vi "Comm String Flush Port.vi"(0 "niDTS Comm Telnet in":refnum<class "niDTS Comm Telnet.lvclass">, 7 "Read Data (F)":bool, 9 "Log Data (F)":bool, 11 "error in (no error)":errorcluster) -> (4 "niDTS Comm Telnet out":refnum<class "niDTS Comm Telnet.lvclass">, 8 "Read Data":string, 15 "error out":errorcluster)   [LabVIEW 2015, in "niDTS CommLib.lvlib" / "niDTS Comm Telnet.lvclass"]
uses:
  niDTS Comm Telnet.lvclass
  Utility/telnet/NI_InternetTK_Core_VIs.lvlib
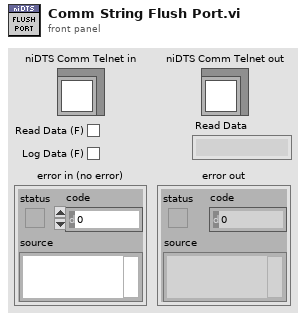
[diagram p1: front panel]
types:
  T1 = typedef "Telnet Session.ctl" = refnum<k1>
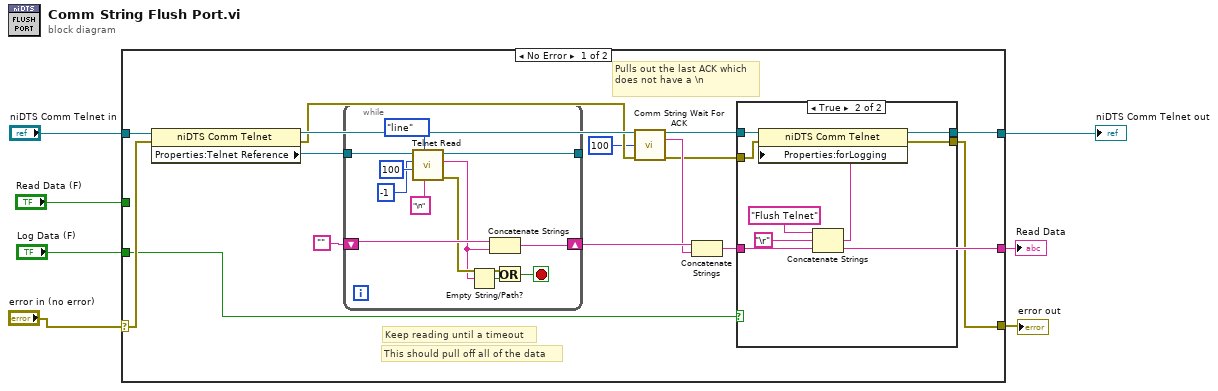
[diagram p0: block diagram]
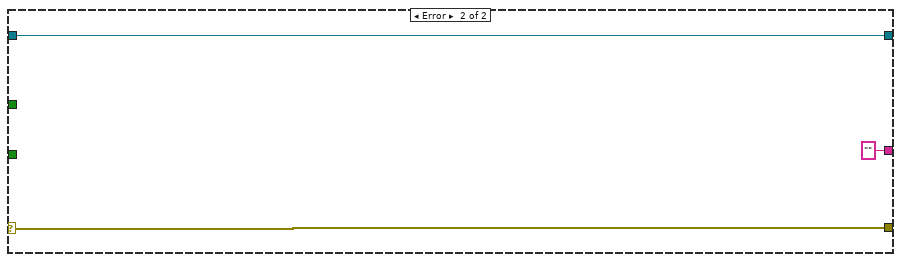
[diagram p3: hidden frame]
diagram:
  n1 = case shown="No Error" "error in (no error)" {
    selector: "error in (no error)" -> [w21 w46]
    tunnel: "niDTS Comm Telnet in" -> [w22 w47]
    tunnel: "Log Data (F)" -> [w11 _]
    tunnel: [w10 w47] -> w3
    tunnel: [w9 w46] -> w1
    tunnel: [w13 ""] -> w2
    tunnel: "Read Data (F)" -> [_ _]
    frame No Error {
      # "Pulls out the last ACK which does not have a \\n"
      # "This should pull off all of the data"
      # "Keep reading until a timeout"
      n2 = property class="niDTS Comm Telnet"(reference=w22, error in=w21) -> (reference out=w18:refnum<class "niDTS Comm Telnet.lvclass">, error out=w17:errorcluster, "Properties:Telnet Reference"=w20:T1)
      n3 = while {
        tunnel: w20 -> [w40]
        shift-right: [w39] -> w16
        shift-left: "" -> [w38]
        tunnel: [w33] -> _
        stop <- w36 stop-if-true
        n4 = call "Telnet Read.vi"("line separator"="\n", "read mode (normal)"=enum16{"normal", "line", "buffered"}."line", "timeout ms (25000)"=100, "bytes to read"=-1, "telnet connection"=w40) -> ("error out"=w35:errorcluster, "data out"=w34:string, "telnet connection out"=w33:T1)  [unwired: 2 in]
        n5 = Empty String/Path?(string/path=w34) -> (empty?=w37:bool)
        n6 = Concatenate Strings(w38, w34) -> (w39:string)
        n7 = Or(x=w35, y=w37) -> (x .or. y?=w36:bool)
      }
      n8 = call-dynamic "Comm String Wait For ACK.vi"("niDTS Comm Telnet in"=w18, "Timeout (ms)"=100, "error in (no error)"=w17) -> ("niDTS Comm Telnet out"=w14:refnum<class "niDTS Comm Telnet.lvclass">, "Response"=w15:string, "error out"=w12:errorcluster)  [unwired: 9 in, 1 out]
      n9 = Concatenate Strings(w16, w15) -> (w13:string)
      n10 = case shown="True" w11 {
        tunnel: w14 -> [w24 w32]
        tunnel: w13 -> [_ w28]
        tunnel: w12 -> [w23 w31]
        tunnel: [w24 w30] -> w10
        tunnel: [w23 w29] -> w9
        frame False {
        }
        frame True {
          n11 = Concatenate Strings("Flush Telnet", "\r", w28) -> (w25:string)
          n12 = property class="niDTS Comm Telnet"(reference=w32, error in=w31, "Properties:forLogging"=w25) -> (reference out=w30:refnum<class "niDTS Comm Telnet.lvclass">, error out=w29:errorcluster)
        }
      }
    }
    frame Error {
    }
  }
  "error out" <- w1
  "niDTS Comm Telnet out" <- w3
  "Read Data" <- w2
